vi "Get All Subscribers.vi"(8 "error in (no error)":errorcluster, 11 "Subscriber Look Up Table in":refnum<class "Subscriber Look Up Table.lvclass">) -> (0 "error out":errorcluster, 2 "Subscribers":refnum<class "Message Transport Interface.lvclass">[](array[class]), 3 "Subscriber Look Up Table out":refnum<class "Subscriber Look Up Table.lvclass">)   [LabVIEW 2016, in "Stream Mediator.lvlib" / "Subscriber Look Up Table.lvclass"]
doc: "--\nCopyright © 2017 Composed SystemsI All rights reserved.\n\nAuthor: Jon McBee <jon.mcbee@composed.io>\n\nThis library is provided \"AS IS\" ,WITHOUT WARRANTIES OR\nCONDITIONS OF ANY KIND, either express or implied.\n\nComposed Systems -- composed.io\n\nStream 0.0.1.1\nJon McBee - Composed Systems\nCopyright (c) 2017, Composed Systems"
uses:
  <userlib>/Composed Systems/Stream/Mediator/Classes/Subscriber Look Up Table/Subscriber Look Up Table.lvclass
  C:/Program Files (x86)/National Instruments/LabVIEW 2016/user.lib/Composed Systems/Stream/Look Up Table/Look Up Table/Look Up Table.lvclass
  <userlib>/Composed Systems/Stream/Mediator/Classes/Message Transport Interface/Message Transport Interface.lvclass
  <userlib>/Composed Systems/Stream/Look Up Table/Look Up Table/Look Up Table.lvclass
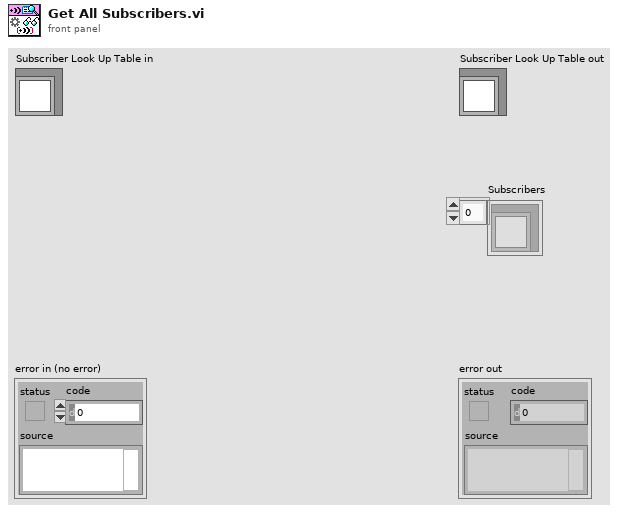
[diagram p1: front panel]
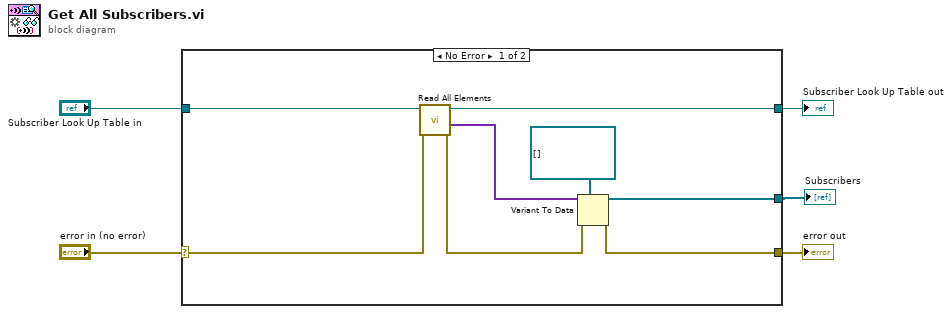
[diagram p0: block diagram]
diagram:
  n1 = case shown="No Error" "error in (no error)" {
    selector: "error in (no error)" -> [w8 w15]
    tunnel: [w11 w15] -> w4
    tunnel: [w9 w14] -> w2
    tunnel: "Subscriber Look Up Table in" -> [w10 w14]
    tunnel: [w12 _] -> w1
    frame No Error {
      n2 = call <userlib>:"Read All Elements.vi"("error in (no error)"=w8, "Look Up Table in"=w10) -> ("error out"=w7:errorcluster, "All Elements"=w6:variant[], "Look Up Table out"=w9:refnum<class "Subscriber Look Up Table.lvclass">)  [unwired: 6 in, 1 out]
      n3 = Variant To Data(error in=w7, type=refnum<class "Message Transport Interface.lvclass">[] [] ("Subscribers"), Variant=w6) -> (data=w12:refnum<class "Message Transport Interface.lvclass">[], error out=w11:errorcluster)
    }
    frame Error {
    }
  }
  "error out" <- w4
  "Subscriber Look Up Table out" <- w2
  "Subscribers" <- w1
